vi "help_pdfs_adq.vi"() -> ()   [LabVIEW 2019]
panel:
  in  "TelasWebServerSensorAD":bool
  in  "Bocal Sônico":bool
  in  "Sonda agulha":bool
  in  "Sonda impedância":bool
  in  "Calibração Corioli":bool
  in  "viscosidade em golfadas":bool
  in  "modelo de filme":bool
  in  "Annual review slug flow Fabre":bool
  in  "golfadas Taitel":bool
  in  "celula Taitel":bool
  in  "Coreeq":bool
  in  "Calibração Placa de orifício":bool
  in  "stop":bool
  in  "Caixa de conexão 2":bool
  in  "Caixa de conexão 1":bool
  in  "Calibração Trans. Pressão seção de teste":bool
  in  "Calibração Elemento de fluxo laminar":bool
  in  "Método Gravimétrico de F  Vazio":bool
  in  "Sensor Anel dissertação Bruno":bool
  in  "Sensor Haste Calibração":bool
  in  "Sensor Haste (2)":bool
  in  "Sensor Anel Artigo":bool
  in  "Sensor Haste (1)":bool
  in  "Sonda elétrica (agulha)":bool
  in  "Técnicas Experimentais":bool
  in  "Processamento Sinais Prog Slug":bool
  in  "Manual Prog Slug":bool
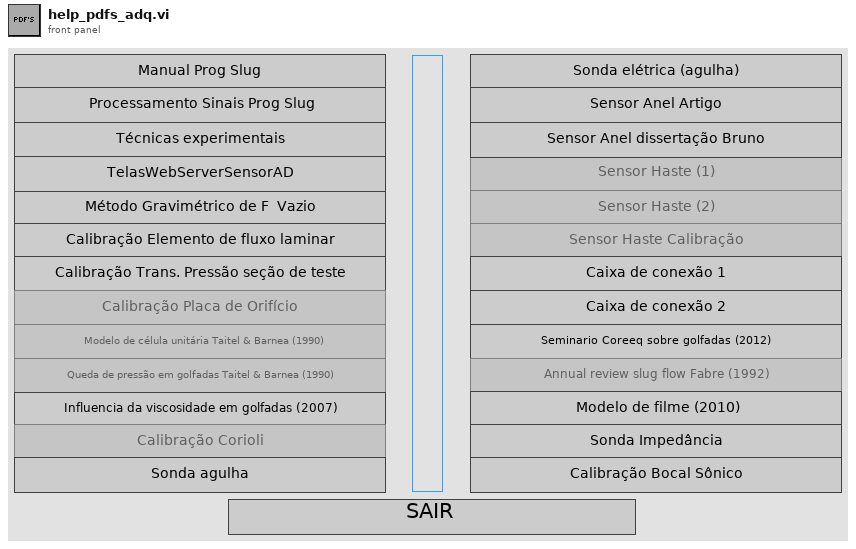
[diagram p1: front panel]
types:
  T1 = enum8{"Enabled", "Disabled", "Disabled and Grayed Out"}
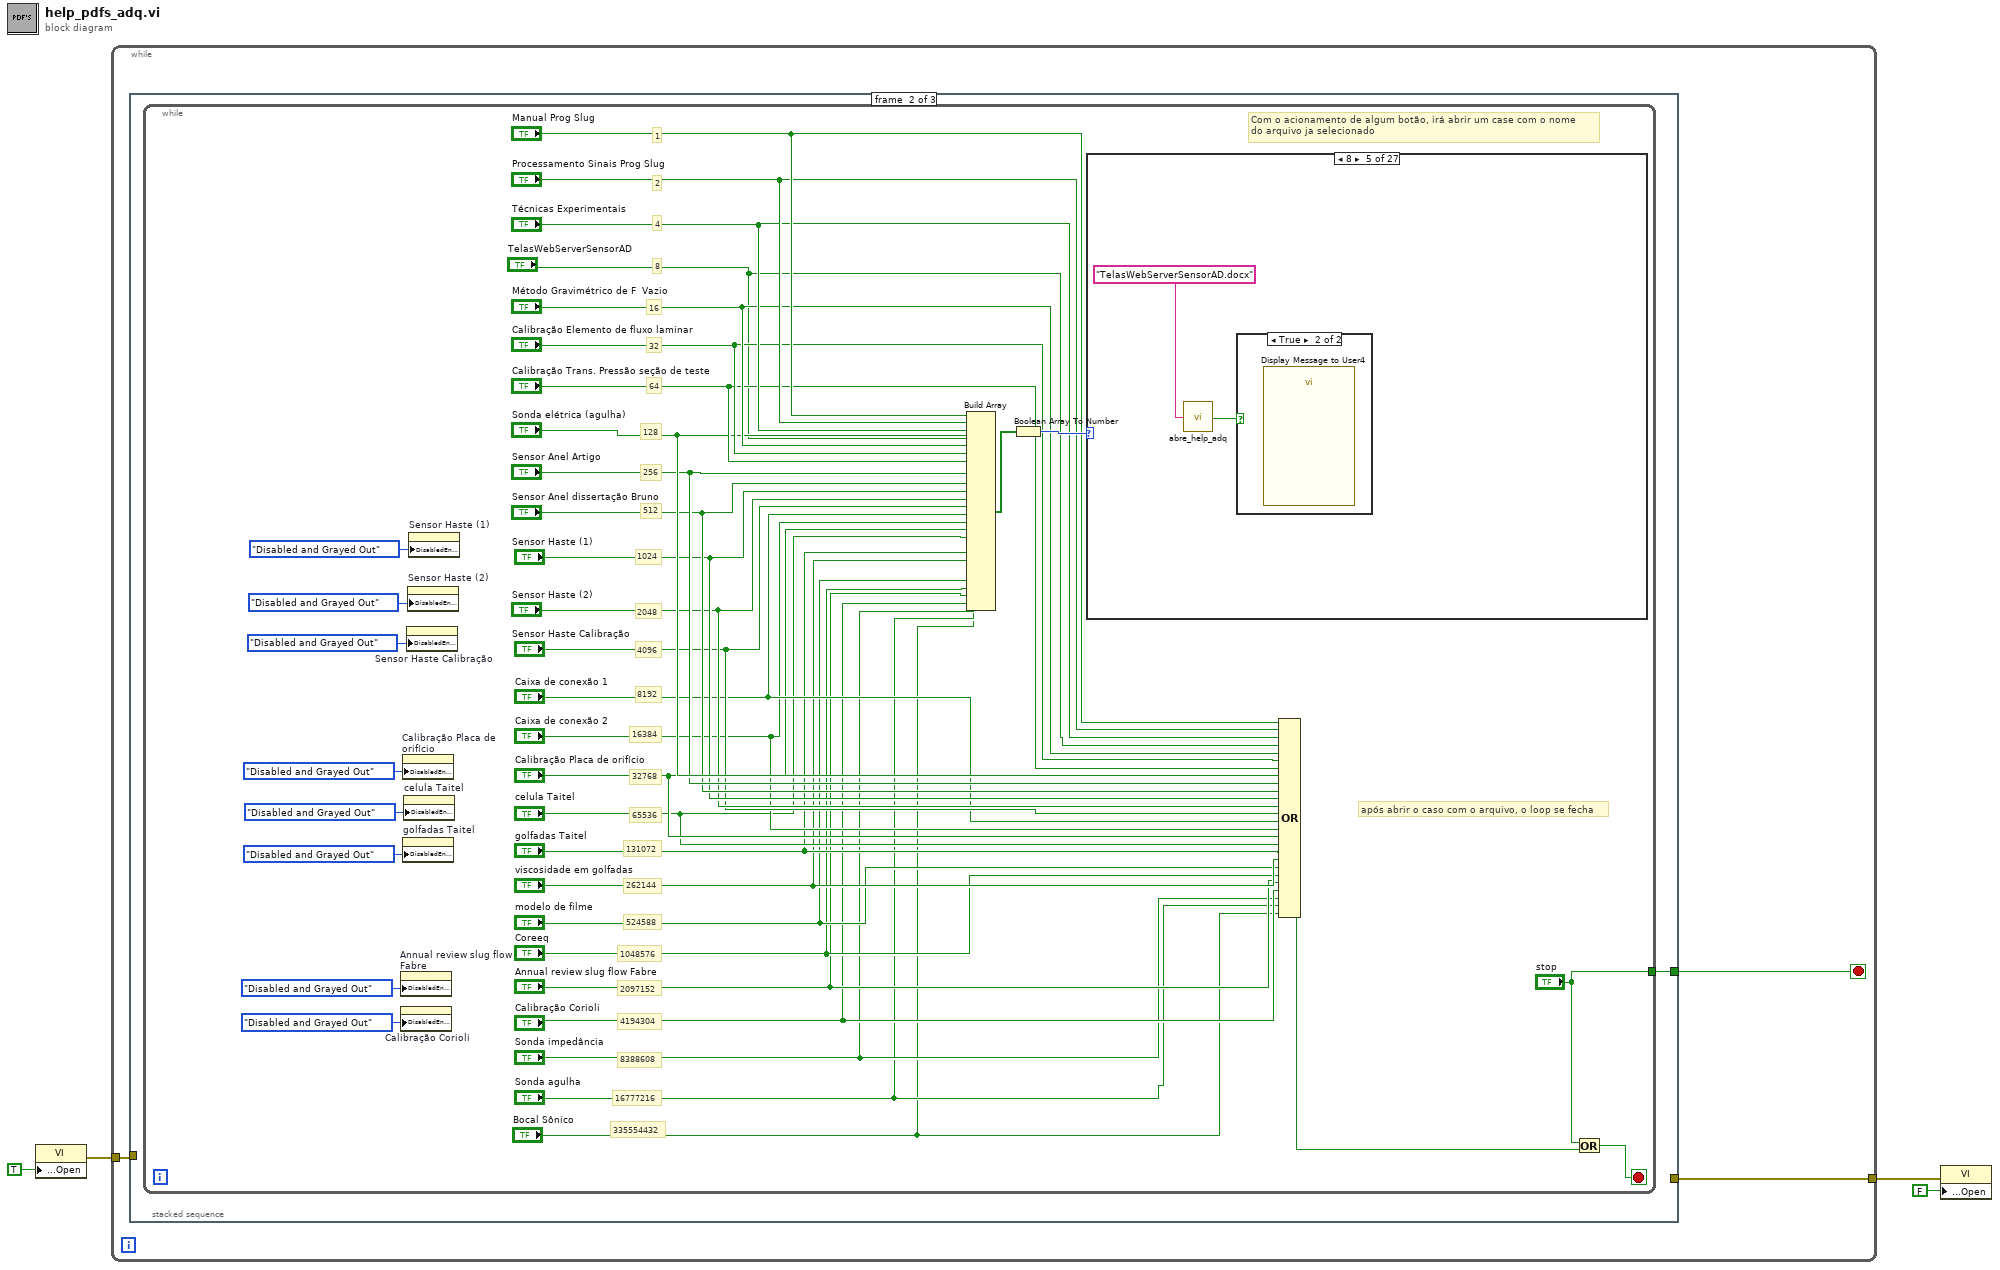
[diagram p0: block diagram]
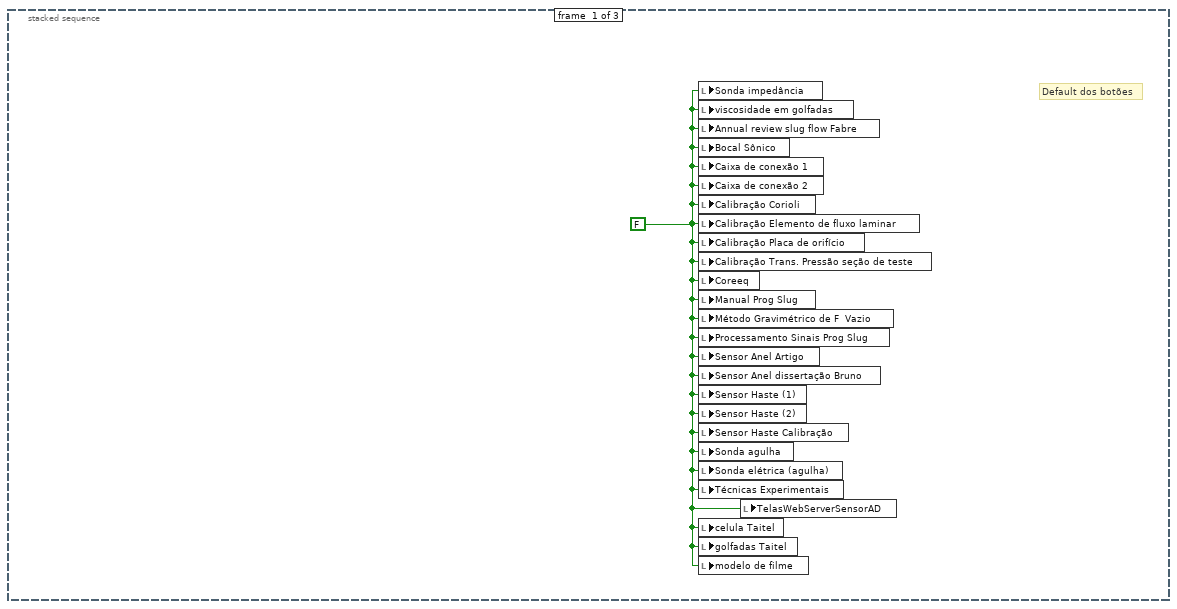
[diagram p2: hidden frame]
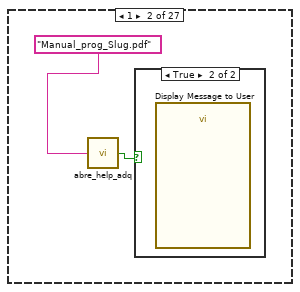
[diagram p4: hidden frame]
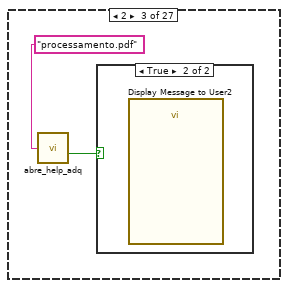
[diagram p6: hidden frame]
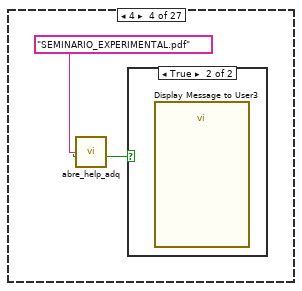
[diagram p8: hidden frame]
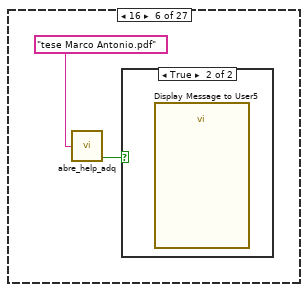
[diagram p11: hidden frame]
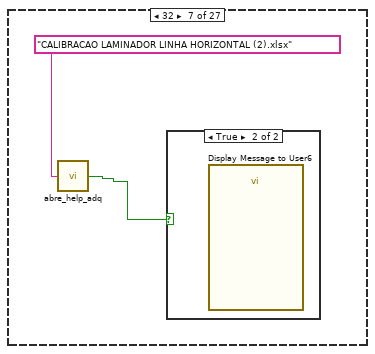
[diagram p13: hidden frame]
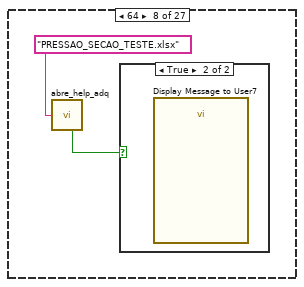
[diagram p15: hidden frame]
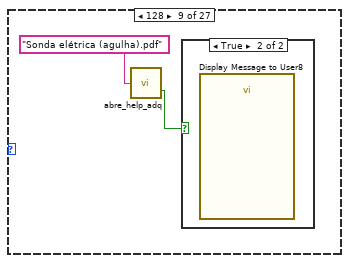
[diagram p17: hidden frame]
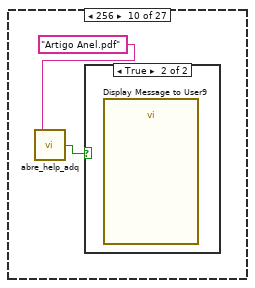
[diagram p19: hidden frame]
diagram:
  n1 = property class="VI"("Front Panel.Open"=TRUE ("Front Panel Window:Open")) -> (error out=w1:errorcluster)  [unwired: 2 in, 1 out]
  n2 = while {
    tunnel: [w6] -> w2
    tunnel: w1 -> [w5]
    stop <- w7 stop-if-true
    n3 = stacked-sequence {
      tunnel: [_ w9 _] -> w7
      tunnel: w5 -> [_ _ w103]
      tunnel: [_ _ w103] -> w6
      frame #0 {
        w8 = FALSE ("Caixa de conexão 1")
        # "Default dos botões"
        n4 = local write "Sonda impedância"(w8) -> ()
        n5 = local write "viscosidade em golfadas"(w8) -> ()
        n6 = local write "Annual review slug flow Fabre"(w8) -> ()
        n7 = local write "Bocal Sônico"(w8) -> ()
        n8 = local write "Caixa de conexão 1"(w8) -> ()
        n9 = local write "Caixa de conexão 2"(w8) -> ()
        n10 = local write "Calibração Corioli"(w8) -> ()
        n11 = local write "Calibração Elemento de fluxo laminar"(w8) -> ()
        n12 = local write "Calibração Placa de orifício"(w8) -> ()
        n13 = local write "Calibração Trans. Pressão seção de teste"(w8) -> ()
        n14 = local write "Coreeq"(w8) -> ()
        n15 = local write "Manual Prog Slug"(w8) -> ()
        n16 = local write "Método Gravimétrico de F  Vazio"(w8) -> ()
        n17 = local write "Processamento Sinais Prog Slug"(w8) -> ()
        n18 = local write "Sensor Anel Artigo"(w8) -> ()
        n19 = local write "Sensor Anel dissertação Bruno"(w8) -> ()
        n20 = local write "Sensor Haste (1)"(w8) -> ()
        n21 = local write "Sensor Haste (2)"(w8) -> ()
        n22 = local write "Sensor Haste Calibração"(w8) -> ()
        n23 = local write "Sonda agulha"(w8) -> ()
        n24 = local write "Sonda elétrica (agulha)"(w8) -> ()
        n25 = local write "Técnicas Experimentais"(w8) -> ()
        n26 = local write "celula Taitel"(w8) -> ()
        n27 = local write "golfadas Taitel"(w8) -> ()
        n28 = local write "modelo de filme"(w8) -> ()
        n29 = local write "TelasWebServerSensorAD"(w8) -> ()
      }
      frame #1 {
        n30 = while {
          tunnel: ["stop"] -> w9
          stop <- w38 stop-if-true
          # "após abrir o caso com o arquivo, o loop se fecha"
          # "Com o acionamento de algum botão, irá abrir um case com o nome \ndo arquivo ja selecionado"
          # "335554432"
          # "16777216"
          # "8388608"
          # "4194304"
          # "2097152"
          # "1048576"
          # "524588"
          # "262144"
          # "131072"
          # "65536"
          # "32768"
          # "16384"
          # "8192"
          # "4096"
          # "2048"
          # "1024"
          # "512"
          # "256"
          # "128"
          # "64"
          # "32"
          # "16"
          # "8"
          # "4"
          # "2"
          # "1"
          n31 = property on="Annual review slug flow Fabre" class="Bool (strict)"("DisabledEnum"=T1."Disabled and Grayed Out" ("Disabled")) -> ()  [unwired: 2 in, 2 out]
          n32 = property on="Calibração Corioli" class="Bool (strict)"("DisabledEnum"=T1."Disabled and Grayed Out" ("Disabled")) -> ()  [unwired: 2 in, 2 out]
          n33 = property on="Calibração Placa de orifício" class="Bool (strict)"("DisabledEnum"=T1."Disabled and Grayed Out" ("Disabled")) -> ()  [unwired: 2 in, 2 out]
          n34 = property on="golfadas Taitel" class="Bool (strict)"("DisabledEnum"=T1."Disabled and Grayed Out" ("Disabled")) -> ()  [unwired: 2 in, 2 out]
          n35 = property on="celula Taitel" class="Bool (strict)"("DisabledEnum"=T1."Disabled and Grayed Out" ("Disabled")) -> ()  [unwired: 2 in, 2 out]
          n36 = property on="Sensor Haste Calibração" class="Bool (strict)"("DisabledEnum"=T1."Disabled and Grayed Out" ("Disabled")) -> ()  [unwired: 2 in, 2 out]
          n37 = property on="Sensor Haste (2)" class="Bool (strict)"("DisabledEnum"=T1."Disabled and Grayed Out" ("Disabled")) -> ()  [unwired: 2 in, 2 out]
          n38 = property on="Sensor Haste (1)" class="Bool (strict)"("DisabledEnum"=T1."Disabled and Grayed Out" ("Disabled")) -> ()  [unwired: 2 in, 2 out]
          n39 = Build Array("Manual Prog Slug", "Processamento Sinais Prog Slug", "Técnicas Experimentais", "TelasWebServerSensorAD", "Método Gravimétrico de F  Vazio", "Calibração Elemento de fluxo laminar", "Calibração Trans. Pressão seção de teste", "Sonda elétrica (agulha)", "Sensor Anel Artigo", "Sensor Anel dissertação Bruno", "Sensor Haste (1)", "Sensor Haste (2)", "Sensor Haste Calibração", "Caixa de conexão 1", "Caixa de conexão 2", "Calibração Placa de orifício", "celula Taitel", "golfadas Taitel", "viscosidade em golfadas", "modelo de filme", "Coreeq", "Annual review slug flow Fabre", "Calibração Corioli", "Sonda impedância", "Sonda agulha", "Bocal Sônico") -> (w48:bool[])
          n40 = Boolean Array To Number(Boolean array=w48) -> (number=w47:u32)
          n41 = case shown="8" w47 {
            frame 0, Default {
            }
            frame 1 {
              n42 = call "abre_help_adq.vi"("nome"="Manual_prog_Slug.pdf") -> ("Erro"=w49:bool)
              n43 = case shown="True" w49 {
                frame False {
                }
                frame True {
                  n44 = call "Display Message to User"() -> ()  [unwired: 10 in, 2 out]
                }
              }
            }
            frame 2 {
              n45 = call "abre_help_adq.vi"("nome"="processamento.pdf") -> ("Erro"=w51:bool)
              n46 = case shown="True" w51 {
                frame False {
                }
                frame True {
                  n47 = call "Display Message to User2"() -> ()  [unwired: 10 in, 2 out]
                }
              }
            }
            frame 4 {
              n48 = call "abre_help_adq.vi"("nome"="SEMINARIO_EXPERIMENTAL.pdf") -> ("Erro"=w53:bool)
              n49 = case shown="True" w53 {
                frame False {
                }
                frame True {
                  n50 = call "Display Message to User3"() -> ()  [unwired: 10 in, 2 out]
                }
              }
            }
            frame 8 {
              n51 = call "abre_help_adq.vi"("nome"="TelasWebServerSensorAD.docx") -> ("Erro"=w55:bool)
              n52 = case shown="True" w55 {
                frame False {
                }
                frame True {
                  n53 = call "Display Message to User4"() -> ()  [unwired: 10 in, 2 out]
                }
              }
            }
            frame 16 {
              n54 = call "abre_help_adq.vi"("nome"="tese Marco Antonio.pdf") -> ("Erro"=w57:bool)
              n55 = case shown="True" w57 {
                frame False {
                }
                frame True {
                  n56 = call "Display Message to User5"() -> ()  [unwired: 10 in, 2 out]
                }
              }
            }
            frame 32 {
              n57 = call "abre_help_adq.vi"("nome"="CALIBRACAO LAMINADOR LINHA HORIZONTAL (2).xlsx") -> ("Erro"=w59:bool)
              n58 = case shown="True" w59 {
                frame False {
                }
                frame True {
                  n59 = call "Display Message to User6"() -> ()  [unwired: 10 in, 2 out]
                }
              }
            }
            frame 64 {
              n60 = call "abre_help_adq.vi"("nome"="PRESSAO_SECAO_TESTE.xlsx") -> ("Erro"=w61:bool)
              n61 = case shown="True" w61 {
                frame False {
                }
                frame True {
                  n62 = call "Display Message to User7"() -> ()  [unwired: 10 in, 2 out]
                }
              }
            }
            frame 128 {
              n63 = call "abre_help_adq.vi"("nome"="Sonda elétrica (agulha).pdf") -> ("Erro"=w63:bool)
              n64 = case shown="True" w63 {
                frame False {
                }
                frame True {
                  n65 = call "Display Message to User8"() -> ()  [unwired: 10 in, 2 out]
                }
              }
            }
            frame 256 {
              n66 = call "abre_help_adq.vi"("nome"="Artigo Anel.pdf") -> ("Erro"=w65:bool)
              n67 = case shown="True" w65 {
                frame False {
                }
                frame True {
                  n68 = call "Display Message to User9"() -> ()  [unwired: 10 in, 2 out]
                }
              }
            }
            frame 512 {
              n69 = call "abre_help_adq.vi"("nome"="Dissertação Bruno.pdf") -> ("Erro"=w67:bool)
              n70 = case shown="True" w67 {
                frame False {
                }
                frame True {
                  n71 = call "Display Message to User10"() -> ()  [unwired: 10 in, 2 out]
                }
              }
            }
            frame 1024 {
              # "nao tem"
              n72 = call "abre_help_adq.vi"("nome"="Haste 1.pdf") -> ("Erro"=w69:bool)
              n73 = case shown="True" w69 {
                frame False {
                }
                frame True {
                  n74 = call "Display Message to User11"() -> ()  [unwired: 10 in, 2 out]
                }
              }
            }
            frame 2048 {
              # "nao tem"
              n75 = call "abre_help_adq.vi"("nome"="Haste 2.pdf") -> ("Erro"=w71:bool)
              n76 = case shown="True" w71 {
                frame False {
                }
                frame True {
                  n77 = call "Display Message to User12"() -> ()  [unwired: 10 in, 2 out]
                }
              }
            }
            frame 4096 {
              # "nao tem"
              n78 = call "abre_help_adq.vi"("nome"="Calibração Haste.xlsx") -> ("Erro"=w73:bool)
              n79 = case shown="True" w73 {
                frame False {
                }
                frame True {
                  n80 = call "Display Message to User13"() -> ()  [unwired: 10 in, 2 out]
                }
              }
            }
            frame 8192 {
              n81 = call "abre_help_adq.vi"("nome"="Black Box - Conexões.pdf") -> ("Erro"=w75:bool)
              n82 = case shown="True" w75 {
                frame False {
                }
                frame True {
                  n83 = call "Display Message to User14"() -> ()  [unwired: 10 in, 2 out]
                }
              }
            }
            frame 16384 {
              n84 = call "abre_help_adq.vi"("nome"="Caixa de conexões.pdf") -> ("Erro"=w77:bool)
              n85 = case shown="True" w77 {
                frame False {
                }
                frame True {
                  n86 = call "Display Message to User15"() -> ()  [unwired: 10 in, 2 out]
                }
              }
            }
            frame 32768 {
              # "nao tem"
              n87 = call "abre_help_adq.vi"("nome"="CALIBRAÇÃO PLACA ORIFÍCIO.xlsx") -> ("Erro"=w79:bool)
              n88 = case shown="True" w79 {
                frame False {
                }
                frame True {
                  n89 = call "Display Message to User16"() -> ()  [unwired: 10 in, 2 out]
                }
              }
            }
            frame 65536 {
              # "nao tem"
              n90 = call "abre_help_adq.vi"("nome"="TAITEL BARNEA 1990 - Two-Phase Slug Flow.pdf") -> ("Erro"=w81:bool)
              n91 = case shown="True" w81 {
                frame False {
                }
                frame True {
                  n92 = call "Display Message to User17"() -> ()  [unwired: 10 in, 2 out]
                }
              }
            }
            frame 131072 {
              # "nao tem"
              n93 = call "abre_help_adq.vi"("nome"="1990 Taitel, Y. e Barnea, D. - A consistent approach for calculating pressure drop in inclined sl.pdf") -> ("Erro"=w83:bool)
              n94 = case shown="True" w83 {
                frame False {
                }
                frame True {
                  n95 = call "Display Message to User18"() -> ()  [unwired: 10 in, 2 out]
                }
              }
            }
            frame 262144 {
              n96 = call "abre_help_adq.vi"("nome"="Influencia_Viscosidade.pdf") -> ("Erro"=w85:bool)
              n97 = case shown="True" w85 {
                frame False {
                }
                frame True {
                  n98 = call "Display Message to User19"() -> ()  [unwired: 10 in, 2 out]
                }
              }
            }
            frame 524288 {
              n99 = call "abre_help_adq.vi"("nome"="9fb7ecb9577f18b08d439320121c3013.pdf") -> ("Erro"=w87:bool)
              n100 = case shown="True" w87 {
                frame False {
                }
                frame True {
                  n101 = call "Display Message to User20"() -> ()  [unwired: 10 in, 2 out]
                }
              }
            }
            frame 1048576 {
              n102 = call "abre_help_adq.vi"("nome"="17 COREEQ Introducao Golfadas-Eugenio.pdf") -> ("Erro"=w89:bool)
              n103 = case shown="True" w89 {
                frame False {
                }
                frame True {
                  n104 = call "Display Message to User21"() -> ()  [unwired: 10 in, 2 out]
                }
              }
            }
            frame 2097152 {
              # "no tem"
              n105 = call "abre_help_adq.vi"("nome"="Annual_Review_Fabre.pdf") -> ("Erro"=w91:bool)
              n106 = case shown="True" w91 {
                frame False {
                }
                frame True {
                  n107 = call "Display Message to User22"() -> ()  [unwired: 10 in, 2 out]
                }
              }
            }
            frame 4194304 {
              # "nao tem"
              n108 = call "abre_help_adq.vi"("nome"="Calibração Corioli.xlsx") -> ("Erro"=w93:bool)
              n109 = case shown="True" w93 {
                frame False {
                }
                frame True {
                  n110 = call "Display Message to User23"() -> ()  [unwired: 10 in, 2 out]
                }
              }
            }
            frame 8388608 {
              n111 = call "abre_help_adq.vi"("nome"="Placas de impedancia.pdf") -> ("Erro"=w95:bool)
              n112 = case shown="True" w95 {
                frame False {
                }
                frame True {
                  n113 = call "Display Message to User24"() -> ()  [unwired: 10 in, 2 out]
                }
              }
            }
            frame 16777216 {
              n114 = call "abre_help_adq.vi"("nome"="Sonda elétrica (agulha).pdf") -> ("Erro"=w97:bool)
              n115 = case shown="True" w97 {
                frame False {
                }
                frame True {
                  n116 = call "Display Message to User25"() -> ()  [unwired: 10 in, 2 out]
                }
              }
            }
            frame 33554432 {
              n117 = Wait (ms)(milliseconds to wait=u32 1000) -> ()  [unwired: 1 out]
              n118 = call "abre_help_adq.vi"("nome"="FENANDO-TG-BOCAL SONICO.pdf") -> ("Erro"=w100:bool)
              n119 = case shown="True" w100 {
                frame False {
                }
                frame True {
                  n120 = call "Display Message to User26"() -> ()  [unwired: 10 in, 2 out]
                }
              }
            }
          }
          n121 = Compound Arithmetic op=OR("Manual Prog Slug", "Processamento Sinais Prog Slug", "Técnicas Experimentais", "TelasWebServerSensorAD", "Método Gravimétrico de F  Vazio", "Calibração Elemento de fluxo laminar", "Calibração Trans. Pressão seção de teste", "Sonda elétrica (agulha)", "Sensor Anel Artigo", "Sensor Anel dissertação Bruno", "Sensor Haste (1)", "Sensor Haste (2)", "Sensor Haste Calibração", "Caixa de conexão 1", "Caixa de conexão 2", "Calibração Placa de orifício", "celula Taitel", "golfadas Taitel", "viscosidade em golfadas", "modelo de filme", "Coreeq", "Annual review slug flow Fabre", "Calibração Corioli", "Sonda impedância", "Sonda agulha", "Bocal Sônico") -> (w11:bool)
          n122 = Or(x="stop", y=w11) -> (x .or. y?=w38:bool)
        }
      }
      frame #2 {
        w102 = TRUE ("Sensor Anel dissertação Bruno")
        # "Default dos botões"
        n123 = local write "Sonda impedância"(w102) -> ()
        n124 = local write "viscosidade em golfadas"(w102) -> ()
        n125 = local write "Annual review slug flow Fabre"(w102) -> ()
        n126 = local write "Bocal Sônico"(w102) -> ()
        n127 = local write "Caixa de conexão 1"(w102) -> ()
        n128 = local write "Caixa de conexão 2"(w102) -> ()
        n129 = local write "Calibração Corioli"(w102) -> ()
        n130 = local write "Calibração Elemento de fluxo laminar"(w102) -> ()
        n131 = local write "Calibração Placa de orifício"(w102) -> ()
        n132 = local write "Calibração Trans. Pressão seção de teste"(w102) -> ()
        n133 = local write "Coreeq"(w102) -> ()
        n134 = local write "Manual Prog Slug"(w102) -> ()
        n135 = local write "Método Gravimétrico de F  Vazio"(w102) -> ()
        n136 = local write "Processamento Sinais Prog Slug"(w102) -> ()
        n137 = local write "Sensor Anel Artigo"(w102) -> ()
        n138 = local write "Sensor Anel dissertação Bruno"(w102) -> ()
        n139 = local write "Sensor Haste (1)"(w102) -> ()
        n140 = local write "Sensor Haste (2)"(w102) -> ()
        n141 = local write "Sensor Haste Calibração"(w102) -> ()
        n142 = local write "Sonda agulha"(w102) -> ()
        n143 = local write "Sonda elétrica (agulha)"(w102) -> ()
        n144 = local write "Técnicas Experimentais"(w102) -> ()
        n145 = local write "celula Taitel"(w102) -> ()
        n146 = local write "golfadas Taitel"(w102) -> ()
        n147 = local write "modelo de filme"(w102) -> ()
        n148 = local write "TelasWebServerSensorAD"(w102) -> ()
      }
    }
  }
  n149 = property class="VI"(error in=w2, "Front Panel.Open"=FALSE ("Front Panel Window:Open")) -> ()  [unwired: 1 in, 2 out]
